vi "SpectralProcessor.vi"(5 "Analysis settings":T1={"Norm. smoothing"=6.0, "Norm. phase offset"=0.0, "Piecewise flattening"=0, "Apply spectral\nenvelope"=TRUE, "Level and\nzero phase"=TRUE, "Realign phase"=TRUE, "Envelope width"=1.6893939393939394, "Power threshold"=343.04692863149205, "Phase zeroing\ninterval (cm-1)"=[], "Sample Channel"=0, "Ref Channel"=0} {"Power threshold" scale=10.0..1000.0; "Envelope width" scale=0.25..4.0; "Piecewise flattening" min=0 max=10 step=1; "Norm. smoothing" min=0.0 max=100.0 step=0.1}, 6 "Sample Linescan":dbl[][][][](array[numeric]), 7 "Task":T2=enum."Verify python session", 8 "Reference BB Spectrum":dbl[][][](array[numeric]), 9 "Reference Spectrum":dbl[][][](array[numeric]), 10 "Sample BB Spectrum":dbl[][][](array[numeric]), 11 "Sample Spectrum":dbl[][][](array[numeric])) -> (0 "Python session out":refnum<k35>, 1 "Output healed linescan":dbl[][][][](array[numeric]), 2 "Output normalized linescan":dbl[][][](array[numeric]), 3 "Output spectrum":dbl[][](array[numeric]), 4 "Python error out":errorcluster)   [LabVIEW 2022 SP3]
uses:
  Control_SpectralProcessor.ctl
  Control_SpectralProcessor_SettingsCluser.ctl
  <vilib>/Utility/sysdir.llb/System Directory Type.ctl
panel:
  in  "Blank 4D array":dbl[][][][](array[numeric])
  in  "Blank 3D array":dbl[][][](array[numeric])
  in  "Blank 2D array":dbl[][](array[numeric])
  out "Python executable":path=path "C:/Users/mnopl/anaconda3/python.exe"
  in  "Python module path":path=path "C:/Users/mnopl/Desktop/software/mnOPSuite/PRISM/python/scandelay_FTIR.py"
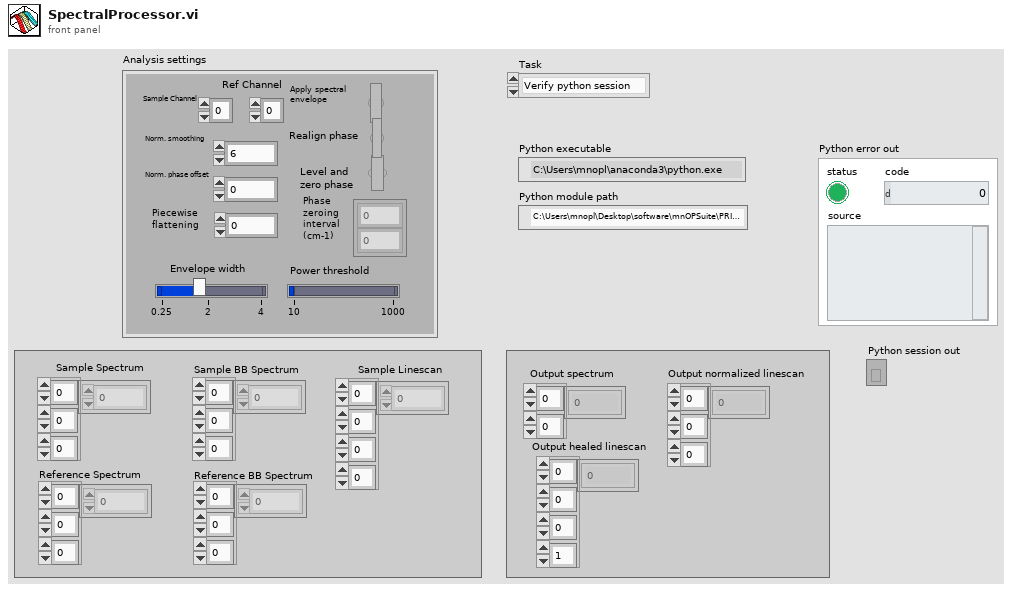
[diagram p1: front panel]
types:
  T1 = typedef "Control_SpectralProcessor_SettingsCluser.ctl" = cluster{"Norm. smoothing":dbl, "Norm. phase offset":dbl, "Piecewise flattening":i16, "Apply spectral\nenvelope":bool, "Level and\nzero phase":bool, "Realign phase":bool, "Envelope width":dbl, "Power threshold":dbl, "Phase zeroing\ninterval (cm-1)":dbl[], "Sample Channel":i32, "Ref Channel":i32}
  T2 = typedef "Control_SpectralProcessor.ctl" = enum16{"Accumulate spectrum", "Verify python session", "Heal linescan", "BB-reference spectrum", "BB-reference linescan", "Normalize spectrum", "Normalize linescan", "Done", "Close python session"}
  T3 = typedef "System Directory Type.ctl" = i32
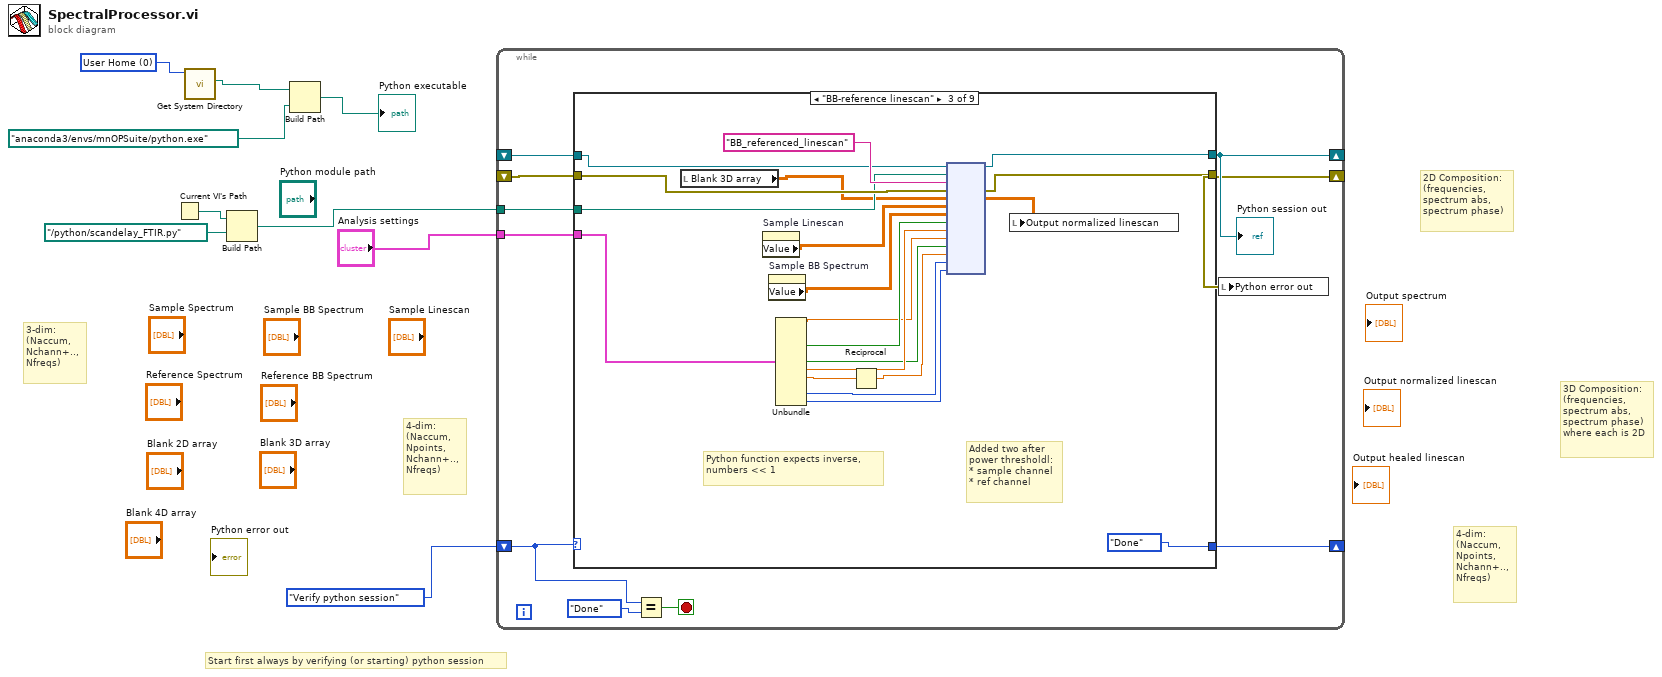
[diagram p0: block diagram]
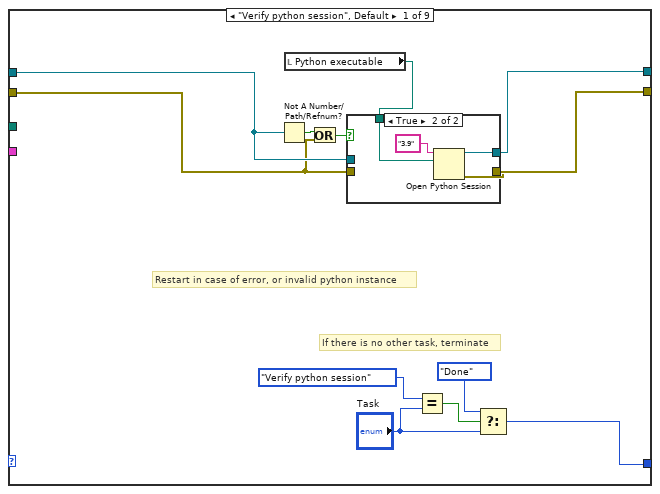
[diagram p2: hidden frame]
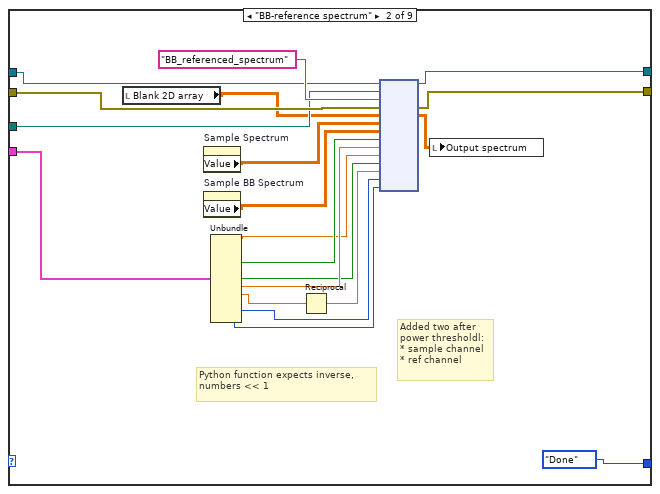
[diagram p4: hidden frame]
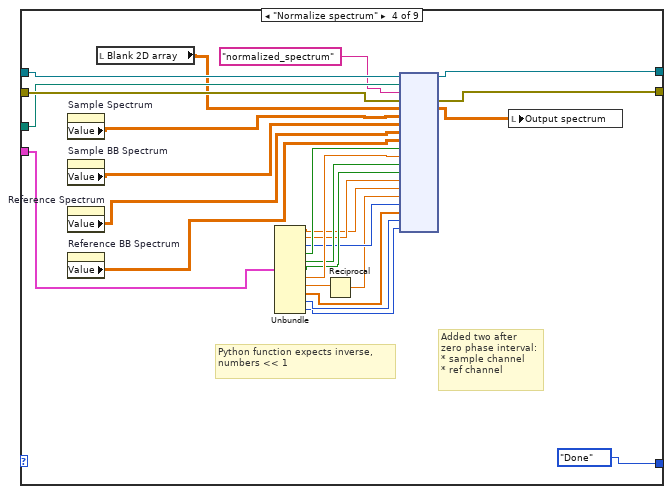
[diagram p5: hidden frame]
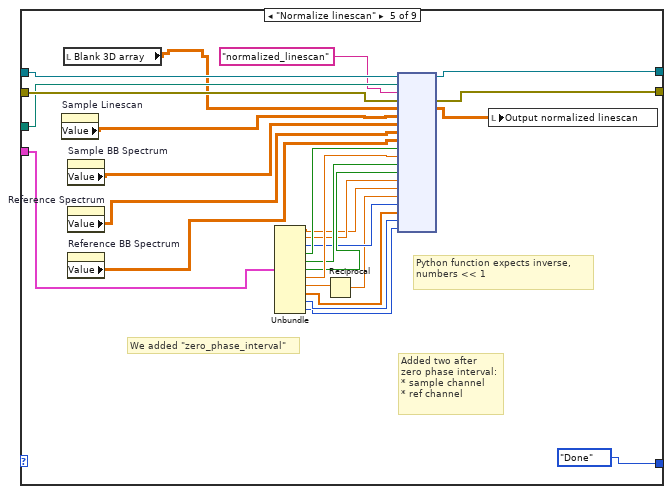
[diagram p6: hidden frame]
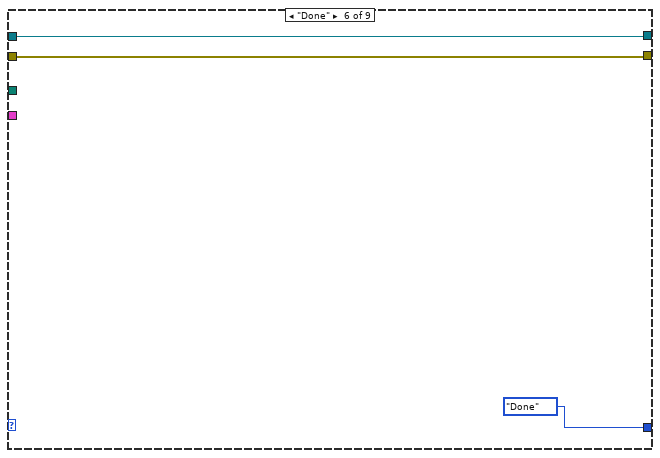
[diagram p7: hidden frame]
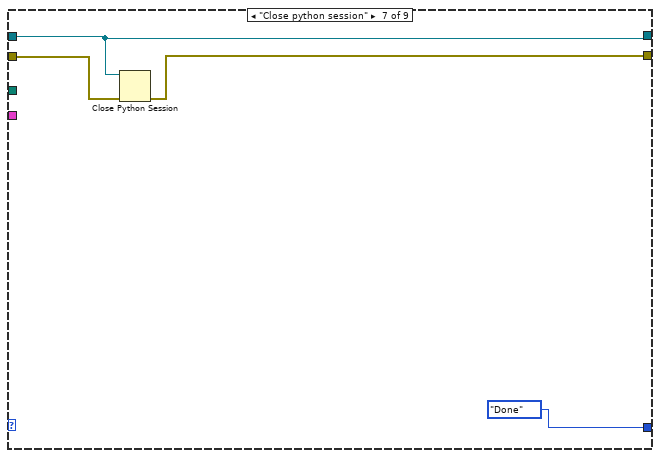
[diagram p8: hidden frame]
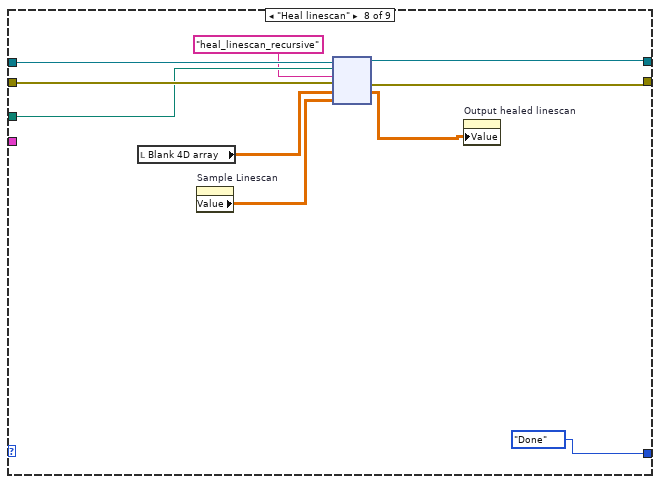
[diagram p9: hidden frame]
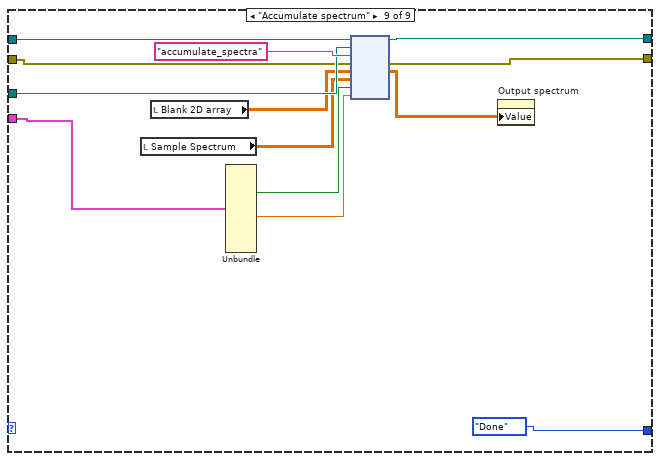
[diagram p10: hidden frame]
diagram:
  w6 = T3 0 items=["User Home"=0, "User Desktop"=1, "User Documents"=2, "User Application Data"=3, "User Preferences"=4, "User Temporary"=5, "Public Documents"=6, "Public Application Data"=7, "Public Preferences"=8, "Public Cache"=13, "System Core Libraries"=9, "System Installed Libraries"=10, "Application Files"=11, "Boot Volume Root"=12] ("system directory type")
  # "4-dim:\n(Naccum,\nNpoints,\nNchann+..,\nNfreqs)"
  # "3D Composition:\n(frequencies,\nspectrum abs,\nspectrum phase)\nwhere each is 2D"
  # "2D Composition:\n(frequencies,\nspectrum abs,\nspectrum phase)"
  # "3-dim:\n(Naccum,\nNchann+..,\nNfreqs)"
  # "4-dim:\n(Naccum,\nNpoints,\nNchann+..,\nNfreqs)"
  # "Start first always by verifying (or starting) python session"
  n1 = Current VI's Path() -> (path=w3:path)
  n2 = call <vilib>:"Get System Directory.vi"("system directory type"=w6) -> ("system directory"=w5:path)  [unwired: 10 in]
  n3 = Build Path(base path=w3, name or relative path=path "../python/scandelay_FTIR.py") -> (appended path=w1:path)
  n4 = Build Path(base path=w5, name or relative path=path "anaconda3/envs/mnOPSuite/python.exe") -> (appended path=→"Python executable":path)
  n5 = while {
    shift-right: [w11] -> _
    shift-left: _ -> [w15]
    shift-right: [w10] -> _
    shift-left: _ -> [w14]
    shift-right: [w18] -> _
    shift-left: Control_SpectralProcessor."Verify python session" -> [w16]
    tunnel: "Analysis settings" -> [w13]
    tunnel: w1 -> [w12]
    stop <- w19 stop-if-true
    n6 = case shown="\"BB-reference linescan\"" w16 {
      tunnel: [w21 Control_SpectralProcessor."Done" Control_SpectralProcessor."Done" Control_SpectralProcessor."Done" Control_SpectralProcessor."Done" Control_SpectralProcessor."Done" Control_SpectralProcessor."Done" Control_SpectralProcessor."Done" Control_SpectralProcessor."Done"] -> w18
      tunnel: w15 -> [w31 w54 w74 w103 w129 w132 w136 w146 w156]
      tunnel: w14 -> [w28 w55 w75 w102 w128 w131 w135 w145 w154]
      tunnel: [w30 w52 w72 w99 w125 w132 w136 w142 w152] -> w11
      tunnel: [w29 w51 w71 w81 w106 w131 w133 w141 w153] -> w10
      tunnel: w13 -> [_ w57 w77 w94 w121 _ _ _ w151]
      tunnel: w12 -> [_ w53 w73 w101 w127 _ _ w144 w155]
      frame "Verify python session", Default {
        # "If there is no other task, terminate"
        # "Restart in case of error, or invalid python instance"
        n7 = Not A Number/Path/Refnum?(number/path/refnum=w31) -> (NaN/Path/Refnum?=w27:bool)
        n8 = local read "Python executable"() -> (w20:path)
        n9 = Or(x=w27, y=w28) -> (x .or. y?=w26:bool)
        n10 = case shown="True" w26 {
          tunnel: [w33 w36] -> w30
          tunnel: [w32 w35] -> w29
          tunnel: w31 -> [w33 _]
          tunnel: w28 -> [w32 _]
          tunnel: w20 -> [_ w34]
          frame False {
          }
          frame True {
            n11 = Open Python Session(python version="3.9", python path=w34) -> (session out=w36:refnum<k35>, error out=w35:errorcluster)  [unwired: 1 in]
          }
        }
        n12 = Equal?(x=Control_SpectralProcessor."Verify python session", y="Task") -> (x = y?=w22:bool)
        n13 = Select(t=Control_SpectralProcessor."Done", s=w22, f="Task") -> (s? t:f=w21:T2)
      }
      frame "BB-reference spectrum" {
        # "Added two after \npower thresholdl:\n* sample channel\n* ref channel"
        # "Python function expects inverse, numbers << 1"
        n14 = local read "Blank 2D array"() -> (w42:dbl[][])
        n15 = property on="Sample Spectrum" class="Arr (strict)"() -> ("Value"=w50:dbl[][][])  [unwired: 2 in, 2 out]
        n16 = property on="Sample BB Spectrum" class="Arr (strict)"() -> ("Value"=w49:dbl[][][])  [unwired: 2 in, 2 out]
        n17 = Unbundle(w57) -> ("Norm. smoothing"=w46:dbl, "Apply spectral\nenvelope"=w48:bool, "Realign phase"=w44:bool, "Envelope width"=w47:dbl, "Power threshold"=w41:dbl, "Sample Channel"=w39:i32, "Ref Channel"=w38:i32)  [unwired: 4 out]
        n18 = Reciprocal(x=w41) -> (1/x=w40:dbl)
        n19 = node(w54, w53, "BB_referenced_spectrum", w55, w42, w50, w49, w48, w47, w46, w44, w40, w39, w38) -> (w52:refnum<k35>, w51:errorcluster, w45:dbl[][])  [unwired: 9 in, 2 out]
        n20 = local write "Output spectrum"(w45) -> ()
      }
      frame "BB-reference linescan" {
        # "Added two after \npower thresholdl:\n* sample channel\n* ref channel"
        # "Python function expects inverse, numbers << 1"
        n21 = local read "Blank 3D array"() -> (w64:dbl[][][])
        n22 = property on="Sample Linescan" class="Arr (strict)"() -> ("Value"=w60:dbl[][][][])  [unwired: 2 in, 2 out]
        n23 = property on="Sample BB Spectrum" class="Arr (strict)"() -> ("Value"=w70:dbl[][][])  [unwired: 2 in, 2 out]
        n24 = Unbundle(w77) -> ("Norm. smoothing"=w67:dbl, "Apply spectral\nenvelope"=w69:bool, "Realign phase"=w66:bool, "Envelope width"=w68:dbl, "Power threshold"=w61:dbl, "Sample Channel"=w59:i32, "Ref Channel"=w58:i32)  [unwired: 4 out]
        n25 = Reciprocal(x=w61) -> (1/x=w62:dbl)
        n26 = node(w74, w73, "BB_referenced_linescan", w75, w64, w60, w70, w69, w68, w67, w66, w62, w59, w58) -> (w72:refnum<k35>, w71:errorcluster, w63:dbl[][][])  [unwired: 9 in, 2 out]
        n27 = local write "Output normalized linescan"(w63) -> ()
      }
      frame "Normalize spectrum" {
        # "Added two after \nzero phase interval:\n* sample channel\n* ref channel"
        # "Python function expects inverse, numbers << 1"
        n28 = property on="Sample Spectrum" class="Arr (strict)"() -> ("Value"=w98:dbl[][][])  [unwired: 2 in, 2 out]
        n29 = property on="Sample BB Spectrum" class="Arr (strict)"() -> ("Value"=w97:dbl[][][])  [unwired: 2 in, 2 out]
        n30 = property on="Reference Spectrum" class="Arr (strict)"() -> ("Value"=w96:dbl[][][])  [unwired: 2 in, 2 out]
        n31 = property on="Reference BB Spectrum" class="Arr (strict)"() -> ("Value"=w95:dbl[][][])  [unwired: 2 in, 2 out]
        n32 = local read "Blank 2D array"() -> (w85:dbl[][])
        n33 = Unbundle(w94) -> ("Norm. smoothing"=w88:dbl, "Norm. phase offset"=w89:dbl, "Piecewise flattening"=w87:i16, "Apply spectral\nenvelope"=w93:bool, "Level and\nzero phase"=w91:bool, "Realign phase"=w90:bool, "Envelope width"=w92:dbl, "Power threshold"=w84:dbl, "Phase zeroing\ninterval (cm-1)"=w80:dbl[], "Sample Channel"=w79:i32, "Ref Channel"=w78:i32)
        n34 = Reciprocal(x=w84) -> (1/x=w83:dbl)
        n35 = node(w103, w101, "normalized_spectrum", w102, w85, w98, w97, w96, w95, w93, w92, w91, w90, w89, w88, w83, w87, w80, w79, w78) -> (w99:refnum<k35>, w81:errorcluster, w82:dbl[][])  [unwired: 15 in, 2 out]
        n36 = local write "Output spectrum"(w82) -> ()
      }
      frame "Normalize linescan" {
        # "Added two after \nzero phase interval:\n* sample channel\n* ref channel"
        # "We added \"zero_phase_interval\""
        # "Python function expects inverse, numbers << 1"
        n37 = property on="Sample Linescan" class="Arr (strict)"() -> ("Value"=w110:dbl[][][][])  [unwired: 2 in, 2 out]
        n38 = local read "Blank 3D array"() -> (w109:dbl[][][])
        n39 = property on="Sample BB Spectrum" class="Arr (strict)"() -> ("Value"=w124:dbl[][][])  [unwired: 2 in, 2 out]
        n40 = property on="Reference Spectrum" class="Arr (strict)"() -> ("Value"=w123:dbl[][][])  [unwired: 2 in, 2 out]
        n41 = property on="Reference BB Spectrum" class="Arr (strict)"() -> ("Value"=w122:dbl[][][])  [unwired: 2 in, 2 out]
        n42 = Unbundle(w121) -> ("Norm. smoothing"=w115:dbl, "Norm. phase offset"=w116:dbl, "Piecewise flattening"=w114:i16, "Apply spectral\nenvelope"=w120:bool, "Level and\nzero phase"=w118:bool, "Realign phase"=w117:bool, "Envelope width"=w119:dbl, "Power threshold"=w112:dbl, "Phase zeroing\ninterval (cm-1)"=w107:dbl[], "Sample Channel"=w105:i32, "Ref Channel"=w104:i32)
        n43 = Reciprocal(x=w112) -> (1/x=w111:dbl)
        n44 = node(w129, w127, "normalized_linescan", w128, w109, w110, w124, w123, w122, w120, w119, w118, w117, w116, w115, w111, w114, w107, w105, w104) -> (w125:refnum<k35>, w106:errorcluster, w108:dbl[][][])  [unwired: 15 in, 2 out]
        n45 = local write "Output normalized linescan"(w108) -> ()
      }
      frame "Done" {
      }
      frame "Close python session" {
        n46 = Close Python Session(session in=w136, error in=w135) -> (11:w133:errorcluster)
      }
      frame "Heal linescan" {
        n47 = local read "Blank 4D array"() -> (w138:dbl[][][][])
        n48 = property on="Sample Linescan" class="Arr (strict)"() -> ("Value"=w139:dbl[][][][])  [unwired: 2 in, 2 out]
        n49 = node(w146, w144, "heal_linescan_recursive", w145, w138, w139) -> (w142:refnum<k35>, w141:errorcluster, w137:dbl[][][][])  [unwired: 1 in, 2 out]
        n50 = property on="Output healed linescan" class="Arr (strict)"("Value"=w137) -> ()  [unwired: 2 in, 2 out]
      }
      frame "Accumulate spectrum" {
        n51 = local read "Sample Spectrum"() -> (w150:dbl[][][])
        n52 = local read "Blank 2D array"() -> (w149:dbl[][])
        n53 = Unbundle(w151) -> ("Apply spectral\nenvelope"=w159:bool, "Envelope width"=w158:dbl)  [unwired: 9 out]
        n54 = node(w156, w155, "accumulate_spectra", w154, w149, w150, w159, w158) -> (w152:refnum<k35>, w153:errorcluster, w148:dbl[][])  [unwired: 3 in, 2 out]
        n55 = property on="Output spectrum" class="Arr (strict)"("Value"=w148) -> ()  [unwired: 2 in, 2 out]
      }
    }
    "Python session out" <- w11
    n56 = Equal?(x=w16, y=Control_SpectralProcessor."Done") -> (x = y?=w19:bool)
    n57 = local write "Python error out"(w10) -> ()
  }
